vi "PDHydra - PWM.vi"(8 "error in":errorcluster, 11 "Board Selector":T1) -> (0 "error out":errorcluster, 1 "0% Duty Cycle":dbl[](array[numeric]), 2 "25% Duty Cycle":dbl[](array[numeric]), 3 "50% Duty Cycle":dbl[](array[numeric]))   [LabVIEW 2022 SP3]
uses:
  Serial Board Com/Board Select.ctl
  HMP4000 Communication/HMP4040_ChannelControl.ctl
  Serial Board Com/ADCSelector BB.ctl
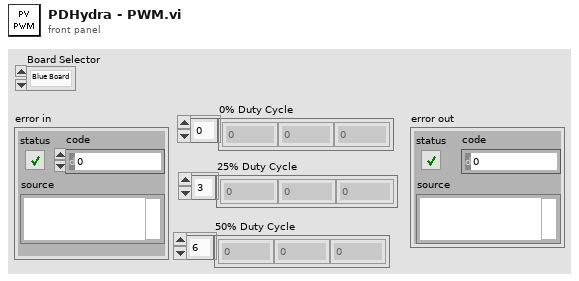
[diagram p1: front panel]
types:
  T1 = typedef "Board Select.ctl" = enum16{"Blue Board", "Green Board"}
  T2 = typedef "HMP4040_ChannelControl.ctl" = cluster{"CH1 Voltage":dbl, "CH1 Current":dbl, "CH1 Output":bool, "CH2 Voltage":dbl, "CH2 Current":dbl, "CH2 Output":bool, "CH3 Voltage":dbl, "CH3 Current":dbl, "CH3 Output":bool, "CH4 Voltage":dbl, "CH4 Current":dbl, "CH4 Output":bool, "Master Output":bool}
  T3 = typedef "ADCSelector BB.ctl" = enum16{"INVA_ISENSE_U", "INVA_ISENSE_V", "INVA_ISENSE_W", "INVA_UDC", "INVA_TEMP", "HB_TEMP", "AUXB_TEMP", "VLINE_AB", "VLINE_BC", "VLINE_CA", "VSENSE_POS_24V", "VSENSE_POS_5V", "VSENSE_NEG_15V", "INVB_ISENSE_U", "INV_B_ISENSEV", "INVB_ISENSE_W", "INVB_UDC", "INVB_TEMP", "AUXA_TEMP", "AUXC_TEMP", "VOUT_AB", "VOUT_BC", "VOUT_CA", "VSENSE_POS_15V", "VSENSE_POS_3P3V", "TEST_POINT"}
  T4 = cluster{"Enum":T3, "Duty Cycle On":i32, "Leg":i32, "Duty Cycle Off":i32}[]
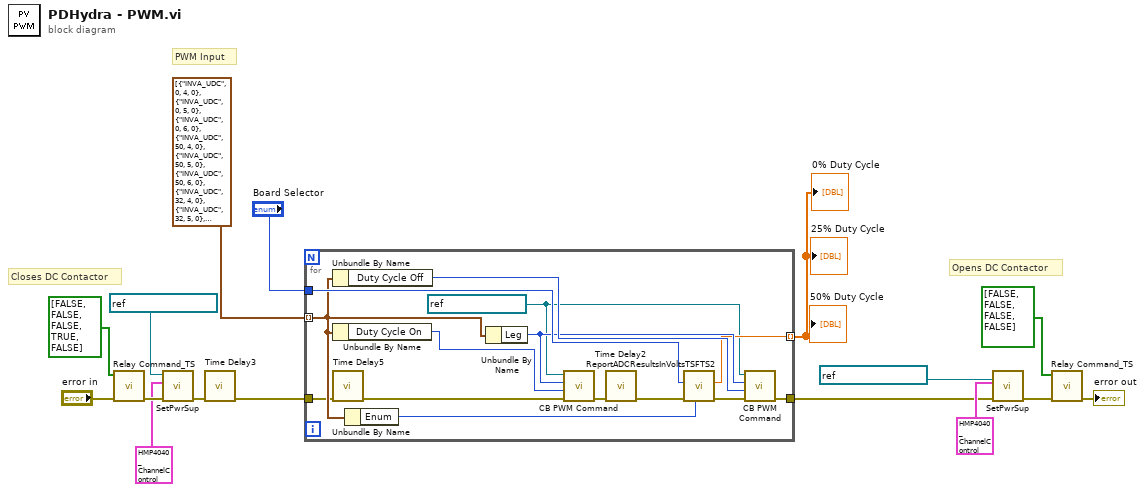
[diagram p0: block diagram]
diagram:
  # "Opens DC Contactor"
  # "PWM Input"
  # "Closes DC Contactor"
  n1 = call "Relay Command_TS.vi"("error in (no error)"="error in", "Relay Command"=bool[] [FALSE, FALSE, FALSE, TRUE, FALSE]) -> ("error out"=w14:errorcluster)  [unwired: 8 in, 1 out]
  n2 = call "SetPwrSup.vi"("error in (no error)"=w14, "HMP4040 Channel Settings"=T2 {"CH1 Voltage"=24.0, "CH1 Current"=1.0, "CH1 Output"=TRUE, "CH2 Voltage"=24.0, "CH2 Current"=5.0, "CH2 Output"=TRUE, "CH3 Voltage"=8.0, "CH3 Current"=1.0, "CH3 Output"=TRUE, "CH4 Voltage"=24.0, "CH4 Current"=1.0, "CH4 Output"=FALSE, "Master Output"=TRUE}, "HMP4040 IN"=refnum<visa-resource-name> "HMP4040_FTS2" ("VISA resource name")) -> ("error out"=w12:errorcluster)  [unwired: 7 in, 1 out]
  n3 = call "Time Delay3"("error in (no error)"=w12) -> ("error out"=w9:errorcluster)  [unwired: 10 in]
  n4 = for {
    tunnel: T4 [{"Enum"=enum."INVA_UDC", "Duty Cycle On"=0, "Leg"=4, "Duty Cycle Off"=0}, {"Enum"=enum."INVA_UDC", "Duty Cycle On"=0, "Leg"=5, "Duty Cycle Off"=0}, {"Enum"=enum."INVA_UDC", "Duty Cycle On"=0, "Leg"=6, "Duty Cycle Off"=0}, {"Enum"=enum."INVA_UDC", "Duty Cycle On"=50, "Leg"=4, "Duty Cycle Off"=0}, {"Enum"=enum."INVA_UDC", "Duty Cycle On"=50, "Leg"=5, "Duty Cycle Off"=0}, {"Enum"=enum."INVA_UDC", "Duty Cycle On"=50, "Leg"=6, "Duty Cycle Off"=0}, {"Enum"=enum."INVA_UDC", "Duty Cycle On"=32, "Leg"=4, "Duty Cycle Off"=0}, {"Enum"=enum."INVA_UDC", "Duty Cycle On"=32, "Leg"=5, "Duty Cycle Off"=0}, {"Enum"=enum."INVA_UDC", "Duty Cycle On"=32, "Leg"=6, "Duty Cycle Off"=0}] -> [w24] mode=indexing
    tunnel: "Board Selector" -> [w29]
    tunnel: [w21] -> w1 mode=indexing
    tunnel: [w20] -> w2
    tunnel: w9 -> [w18]
    w19 = refnum<visa-resource-name> "ControlBoard" ("VISA Refnum in")
    n5 = Unbundle By Name(w24) -> ("Duty Cycle Off"=w23:i32)
    n6 = Unbundle By Name(w24) -> ("Duty Cycle On"=w28:i32)
    n7 = call "Time Delay5"("error in (no error)"=w18) -> ("error out"=w17:errorcluster)  [unwired: 10 in]
    n8 = Unbundle By Name(w24) -> ("Enum"=w30:T3)
    n9 = Unbundle By Name(w24) -> ("Leg"=w22:i32)
    n10 = call "CB PWM Command.vi"("error in (no error)"=w17, "Duty Cycle"=w28, "Leg"=w22, "VISA Refnum in"=w19) -> ("error out"=w27:errorcluster)  [unwired: 5 in, 2 out]
    n11 = call "Time Delay2"("error in (no error)"=w27) -> ("error out"=w26:errorcluster)  [unwired: 10 in]
    n12 = call "ReportADCResultsInVoltsTSFTS2.vi"("Blue Board Enum"=w30, "error in (no error)"=w26, "Board Selector"=w29) -> ("error out"=w25:errorcluster, "Result"=w21:dbl)  [unwired: 5 in, 2 out]
    n13 = call "CB PWM Command.vi"("error in (no error)"=w25, "Duty Cycle"=w23, "Leg"=w22, "VISA Refnum in"=w19) -> ("error out"=w20:errorcluster)  [unwired: 5 in, 2 out]
  }
  "50% Duty Cycle" <- w1
  "25% Duty Cycle" <- w1
  "0% Duty Cycle" <- w1
  n14 = call "SetPwrSup.vi"("error in (no error)"=w2, "HMP4040 Channel Settings"=T2 {"CH1 Voltage"=24.0, "CH1 Current"=1.0, "CH1 Output"=TRUE, "CH2 Voltage"=24.0, "CH2 Current"=5.0, "CH2 Output"=TRUE, "CH3 Voltage"=32.0, "CH3 Current"=1.0, "CH3 Output"=FALSE, "CH4 Voltage"=24.0, "CH4 Current"=1.0, "CH4 Output"=FALSE, "Master Output"=TRUE}, "HMP4040 IN"=refnum<visa-resource-name> "HMP4040_FTS2" ("VISA resource name")) -> ("error out"=w8:errorcluster)  [unwired: 7 in, 1 out]
  n15 = call "Relay Command_TS.vi"("error in (no error)"=w8, "Relay Command"=bool[] [FALSE, FALSE, FALSE, FALSE]) -> ("error out"=→"error out":errorcluster)  [unwired: 8 in, 1 out]
